vi "confirm_function.vi"(10 "Input":i32[][](array[numeric]), 11 "Ring":i32) -> (2 "Boolean 2":bool, 3 "Boolean":bool)   [LabVIEW 2021]
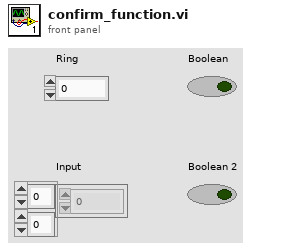
[diagram p1: front panel]
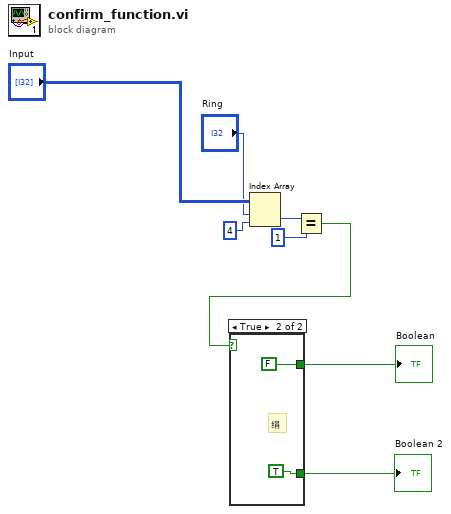
[diagram p0: block diagram]
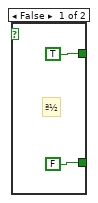
[diagram p2: hidden frame]
diagram:
  n1 = Index Array(array="Input", index (row)="Ring", index (col)=4) -> (element=w3:i32)
  n2 = Equal?(x=w3, y=1) -> (x = y?=w5:bool)
  n3 = case shown="True" w5 {
    tunnel: [FALSE TRUE] -> w7
    tunnel: [TRUE FALSE] -> w8
    frame False {
      # "ª½"
    }
    frame True {
      # "绢"
    }
  }
  "Boolean" <- w8
  "Boolean 2" <- w7
